vi "WPI_JoystickMecanumPolarMapping.vi"(6 "Max Output":dbl=1.0, 8 "Rotation":dbl, 9 "Direction":dbl, 10 "Magnitude":dbl) -> (0 "Rear Right":dbl, 1 "Rear Left":dbl, 2 "Front Right":dbl, 3 "Front Left":dbl)   [LabVIEW 2017]
doc: "Maps the joystick inputs for holonomic driving. Holonomic driving allows you to move the robot in any direction without first rotating or maneuvering the robot.\n\nThis VI assumes the robot to have either four omni-directional wheels and four motors mounted at 45 degree angles in the four corners of a square frame or to have four mecanum wheels driven by four motors."
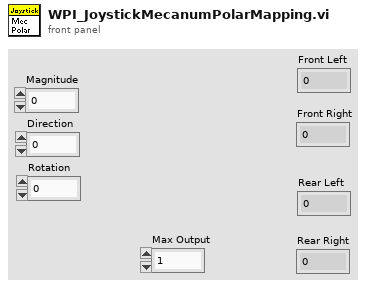
[diagram p1: front panel]
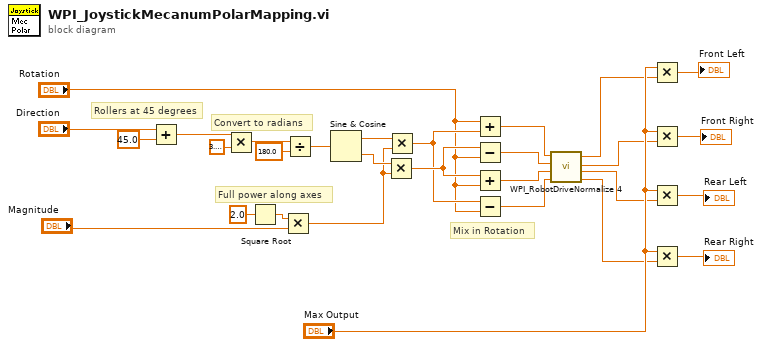
[diagram p0: block diagram]
diagram:
  # "Mix in Rotation"
  # "Convert to radians"
  # "Rollers at 45 degrees"
  # "Full power along axes"
  n1 = Add(x="Direction", y=45.0) -> (x+y=w21:dbl)
  n2 = Multiply(x=w21, y=3.141592653589793) -> (x*y=w19:dbl)
  n3 = Square Root(x=2.0) -> (sqrt(x)=w14:dbl)
  n4 = Multiply(x=w14, y="Magnitude") -> (x*y=w15:dbl)
  n5 = Divide(x=w19, y=180.0) -> (x/y=w27:dbl)
  n6 = Sine & Cosine(0:w27) -> (1:w28:dbl, 2:w29:dbl)
  n7 = Multiply(x=w29, y=w15) -> (x*y=w17:dbl)
  n8 = Multiply(x=w28, y=w15) -> (x*y=w16:dbl)
  n9 = Add(x="Rotation", y=w16) -> (x+y=w23:dbl)
  n10 = Subtract(x=w17, y="Rotation") -> (x-y=w24:dbl)
  n11 = Add(x=w17, y="Rotation") -> (x+y=w25:dbl)
  n12 = Subtract(x=w16, y="Rotation") -> (x-y=w26:dbl)
  n13 = call <vilib>:"WPI_RobotDriveNormalize 4.vi"("D"=w26, "C"=w25, "B"=w24, "A"=w23) -> ("D'"=w5:dbl, "C'"=w6:dbl, "B'"=w7:dbl, "A'"=w8:dbl)
  n14 = Multiply(x="Max Output", y=w8) -> (x*y=→"Front Left":dbl)
  n15 = Multiply(x="Max Output", y=w7) -> (x*y=→"Front Right":dbl)
  n16 = Multiply(x="Max Output", y=w6) -> (x*y=→"Rear Left":dbl)
  n17 = Multiply(x="Max Output", y=w5) -> (x*y=→"Rear Right":dbl)
